vi "exceptions store calling parameters.vi"(7 "levels":u8=1, 11 "exception in":T1 {"code" format="%.0x"}) -> (3 "exception out":T1 {"code" format="%.0x"})   [LabVIEW 2013]
uses:
  exception.ctl
  exception.lvlib
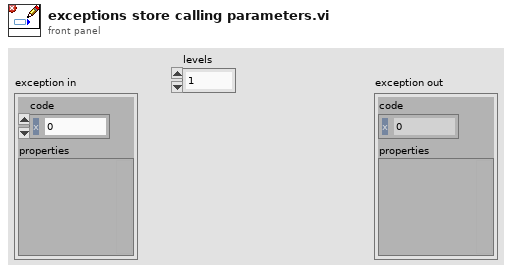
[diagram p1: front panel]
types:
  T1 = typedef "exception.lvlib/exception.ctl" = cluster{"code":i32, "properties":variant}
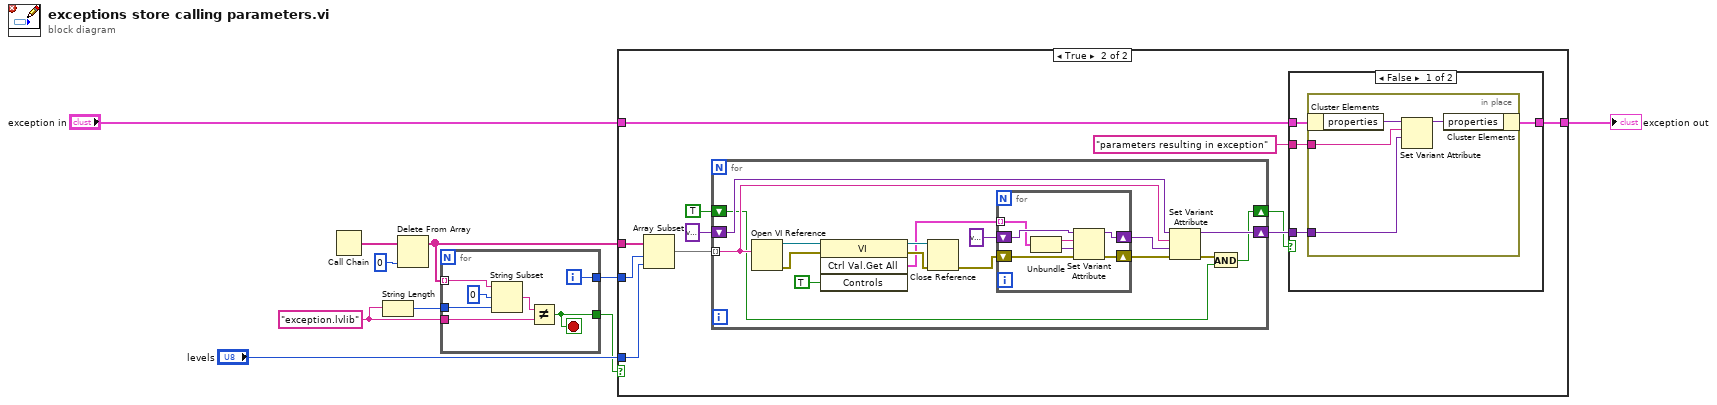
[diagram p0: block diagram]
diagram:
  w6 = "exception.lvlib"
  n1 = Call Chain() -> (call chain=w3:string[])
  n2 = String Length(string=w6) -> (length=w7:i32)
  n3 = Delete From Array(array=w3, index=0) -> (array with subset deleted=w1:string[])  [unwired: 1 in, 1 out]
  n4 = for {
    tunnel: w1 -> [w13] mode=indexing
    tunnel: w7 -> [w17]
    tunnel: w6 -> [w14]
    tunnel: [w12] -> w5
    tunnel: [w11] -> w4
    i -> [w11]
    stop <- w12 stop-if-true
    n5 = String Subset(string=w13, offset (0)=0, length (rest)=w17) -> (substring=w15:string)
    n6 = Not Equal?(x=w15, y=w14) -> (x != y?=w12:bool)
  }
  n7 = case shown="True" w5 {
    tunnel: "exception in" -> [w18 w25]
    tunnel: [w18 w24] -> w10
    tunnel: w1 -> [_ w29]
    tunnel: w4 -> [_ w28]
    tunnel: "levels" -> [_ w27]
    frame False {
    }
    frame True {
      n8 = Array Subset(array=w29, index=w28, length=w27) -> (w26:string[])
      n9 = for {
        shift-right: [w45] -> w22
        shift-left: variant ("name") -> [w44]
        tunnel: w26 -> [w47] mode=indexing
        shift-right: [w41] -> w20
        shift-left: TRUE -> [w40]
        n10 = Open VI Reference(vi path=w47) -> (vi reference=w54:refnum<vi>, error out=w53:errorcluster)  [unwired: 5 in]
        n11 = invoke class="VI" method="Ctrl Val.Get All"(reference=w54, error in=w53, "Controls"=TRUE) -> (reference out=w51:refnum<vi>, error out=w52:errorcluster, "Get All Control Values Variant"=w49:cluster{"Name":string, "Variant Data":variant}[])  [unwired: 1 in, 1 out]
        n12 = Close Reference(reference=w51, error in (no error)=w52) -> (error out=w50:errorcluster)
        n13 = for {
          shift-right: [w60] -> w46
          shift-left: variant ("properties") -> [w61]
          tunnel: w49 -> [w58] mode=indexing
          shift-right: [w55] -> w43
          shift-left: w50 -> [w59]
          n14 = Unbundle(w58) -> ("Name"=w56:string, "Variant Data"=w57:variant)
          n15 = Set Variant Attribute(Variant=w61, name=w56, value=w57, error in=w59) -> (Variant out=w60:variant, error out=w55:errorcluster)  [unwired: 1 out]
        }
        n16 = Set Variant Attribute(Variant=w44, name=w47, value=w46, error in=w43) -> (Variant out=w45:variant, error out=w42:errorcluster)  [unwired: 1 out]
        n17 = And(x=w42, y=w40) -> (x .and. y?=w41:bool)
      }
      n18 = case shown="False" w20 {
        tunnel: w25 -> [w33 w38]
        tunnel: [w32 w38] -> w24
        tunnel: "parameters resulting in exception" ("name") -> [w31 _]
        tunnel: w22 -> [w30 _]
        frame False {
          n19 = in-place {
            in-place-border: w31 -> [w35]
            in-place-border: w30 -> [w34]
            n20 = in-place-cluster #1(w33) -> ("properties"=w36:variant)
            n21 = Set Variant Attribute(Variant=w36, name=w35, value=w34) -> (Variant out=w37:variant)  [unwired: 1 in, 2 out]
            n22 = in-place-cluster #1("properties"=w37) -> (w32:T1)
          }
        }
        frame True {
        }
      }
    }
  }
  "exception out" <- w10
